vi "手动控制.vi"(8 "error in (no error)":errorcluster caption="错误输入（无错误）", 11 "信号灯成员类 输入":refnum<class "信号灯成员类.lvclass">) -> (0 "error out":errorcluster caption="错误输出", 3 "信号灯成员类 输出":refnum<class "信号灯成员类.lvclass">)   [LabVIEW 2017, in "信号灯成员类.lvclass"]
panel:
  in  "状态":enum16{"绿灯亮", "黄灯亮", "红灯亮", "全部亮", "全部熄灭"}(ring)
  in  "关闭":bool
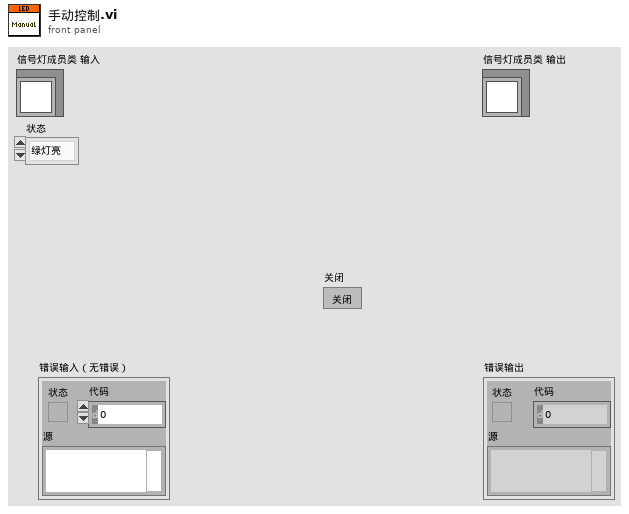
[diagram p1: front panel]
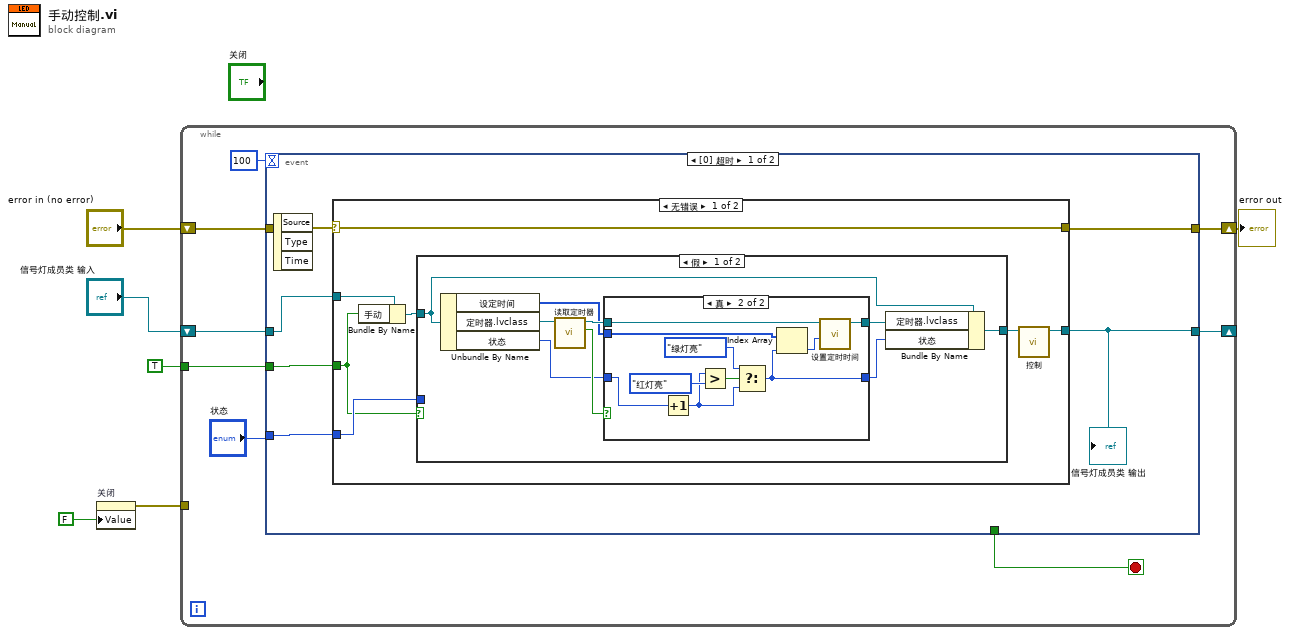
[diagram p0: block diagram]
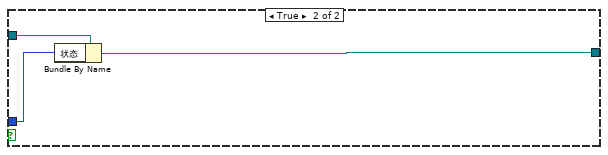
[diagram p3: hidden frame]
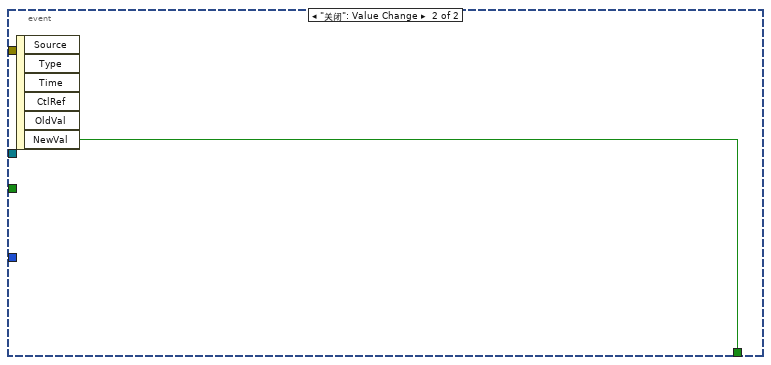
[diagram p5: hidden frame]
diagram:
  n1 = property on="关闭" class="Bool (严格)"("Value"=FALSE ("关闭")) -> (error out=w2:errorcluster)  [unwired: 2 in, 1 out]
  n2 = while {
    tunnel: TRUE ("关闭") -> [w11]
    shift-right: [w13] -> w5
    shift-left: "error in (no error)" -> [w14]
    shift-right: [w9] -> _
    shift-left: "信号灯成员类 输入" -> [w12]
    tunnel: w2 -> [_]
    stop <- w10 stop-if-true
    n3 = event shown="[0] 超时" {
      selector: _ -> [_ _]
      dyn-events: _ -> [_ _]
      timeout: 100 -> [_ _]
      tunnel: w14 -> [w20 _]
      tunnel: [w19 _] -> w13
      tunnel: w12 -> [w18 _]
      tunnel: [w17 _] -> w9
      tunnel: w11 -> [w16 _]
      tunnel: "状态" -> [w15 _]
      tunnel: [_ w54] -> w10
      event Timeout {
        n4 = event-data() -> ()  [unwired: 1 in, 3 out]
        n5 = case shown="无错误" w20 {
          selector: w20 -> [w27 w53]
          tunnel: [w27 w53] -> w19
          tunnel: [w25 w52] -> w17
          tunnel: w18 -> [w26 w52]
          tunnel: w16 -> [w22 _]
          tunnel: w15 -> [w23 _]
          frame No Error {
            n6 = Bundle By Name(cluster=w26, "手动"=w22) -> (w24:refnum<class "信号灯成员类.lvclass">)
            n7 = case shown="假" w22 {
              tunnel: w24 -> [w32 w51]
              tunnel: [w30 w49] -> w21
              tunnel: w23 -> [_ w50]
              frame False {
                n8 = Unbundle By Name(w32) -> ("设定时间"=w33:u32[], "定时器.lvclass"=w36:refnum<class "定时器.lvclass">, "状态"=w28:enum16{"绿灯亮", "黄灯亮", "红灯亮", "全部亮", "全部熄灭"})
                n9 = call "读取定时器.vi"("定时器 输入"=w36) -> ("定时到"=w35:bool, "定时器 输出"=w34:refnum<class "定时器.lvclass">)  [unwired: 1 in, 8 out]
                n10 = case shown="真" w35 {
                  tunnel: w34 -> [w38 w46]
                  tunnel: w33 -> [_ w45]
                  tunnel: [w38 w43] -> w31
                  tunnel: [w37 w40] -> w29
                  tunnel: w28 -> [w37 w39]
                  frame False {
                  }
                  frame True {
                    n11 = Increment(x=w39) -> (x+1=w41:enum16{"绿灯亮", "黄灯亮", "红灯亮", "全部亮", "全部熄灭"})
                    n12 = Greater?(x=w41, y=enum16{"绿灯亮", "黄灯亮", "红灯亮", "全部亮", "全部熄灭"}."红灯亮") -> (0:w47:bool)
                    n13 = Select(t=enum16{"绿灯亮", "黄灯亮", "红灯亮", "全部亮", "全部熄灭"}."绿灯亮" ("y"), s=w47, f=w41) -> (s? t:f=w40:enum16{"绿灯亮", "黄灯亮", "红灯亮", "全部亮", "全部熄灭"})
                    n14 = Index Array(array=w45, index=w40) -> (element=w44:u32)
                    n15 = call-dynamic "设置定时时间.vi"("设置时间"=w44, "定时器 输入"=w46) -> ("定时器 输出"=w43:refnum<class "定时器.lvclass">)  [unwired: 1 in, 8 out]
                  }
                }
                n16 = Bundle By Name(cluster=w32, "定时器.lvclass"=w31, "状态"=w29) -> (w30:refnum<class "信号灯成员类.lvclass">)
              }
              frame True {
                n17 = Bundle By Name(cluster=w51, "状态"=w50) -> (w49:refnum<class "信号灯成员类.lvclass">)
              }
            }
            n18 = call "控制.vi"("信号灯成员类 输入"=w21) -> ("信号灯成员类 输出"=w25:refnum<class "信号灯成员类.lvclass">)  [unwired: 1 in, 9 out]
          }
          frame Error {
          }
        }
        "信号灯成员类 输出" <- w17
      }
      event "关闭": Value Change {
        n19 = event-data() -> ("NewVal"=w54:bool)  [unwired: 1 in, 5 out]
      }
    }
  }
  "error out" <- w5
